vi "Read Connection Ref.vi"(8 "error in (no error)":errorcluster, 11 "Access in":refnum<class "Access.lvclass">) -> (0 "error out":errorcluster, 2 "connection reference":T1, 3 "Access out":refnum<class "Access.lvclass">)   [LabVIEW 2021, in "Database.lvlib" / "Access.lvclass"]
uses:
  Access.lvclass
  <vilib>/addons/database/Connection.llb/Conn ObjectReference.ctl
  Access.lvclass/Access.ctl
  <vilib>/addons/database/NI_Database_API.lvlib
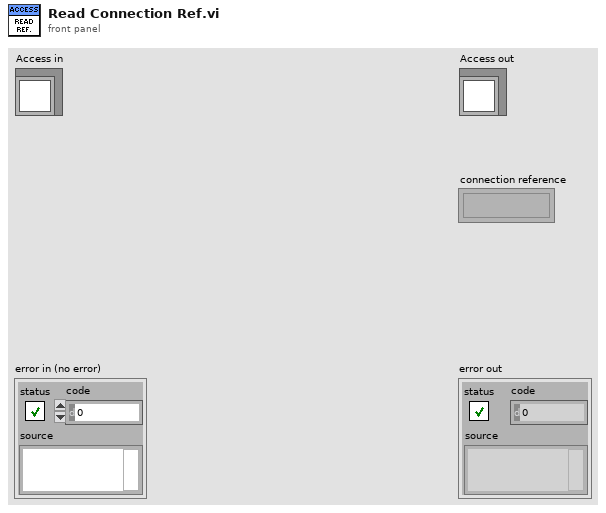
[diagram p1: front panel]
types:
  T1 = typedef "NI_Database_API.lvlib/Conn ObjectReference.ctl" = refnum<k1>
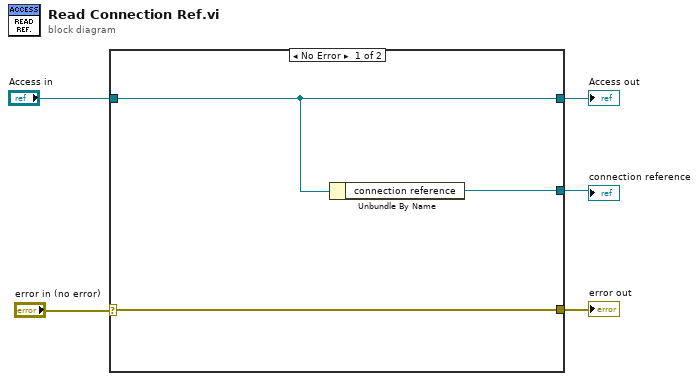
[diagram p0: block diagram]
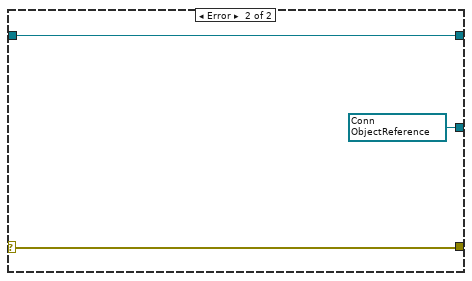
[diagram p2: hidden frame]
diagram:
  n1 = case shown="No Error" "error in (no error)" {
    selector: "error in (no error)" -> [w8 w10]
    tunnel: "Access in" -> [w7 w11]
    tunnel: [w7 w11] -> w3
    tunnel: [w8 w10] -> w2
    tunnel: [w6 w9] -> w1
    frame No Error {
      n2 = Unbundle By Name(w7) -> ("connection reference"=w6:T1)
    }
    frame Error {
      w9 = T1 refnum items=["Connection"] ("connection reference")
    }
  }
  "error out" <- w2
  "Access out" <- w3
  "connection reference" <- w1
